vi "int32 to Hex vg.vi"(11 "number":dbl) -> (1 "Phase fied":string, 3 "E field":string)   [LabVIEW 2017]
panel:
  out "concatenated string both":string
  out "concatenated higher":string
  out "concatenated string lower":string
  out "Hex string":string
  # "RE-ENTRANT"
  # "SUBROUTINE"
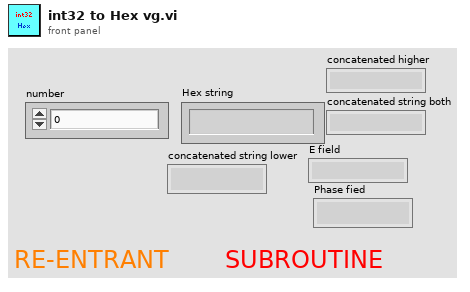
[diagram p1: front panel]
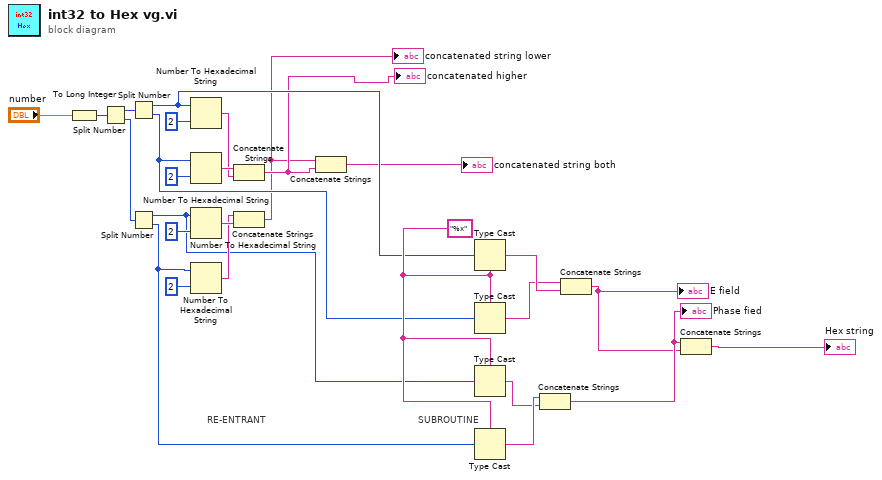
[diagram p0: block diagram]
diagram:
  w15 = "%x" ("type")
  # "SUBROUTINE"
  # "RE-ENTRANT"
  n1 = To Long Integer(number="number") -> (32bit integer=w22:i32)
  n2 = Split Number(x=w22) -> (hi(x)=w26:u16, lo(x)=w27:u16)
  n3 = Split Number(x=w26) -> (hi(x)=w12:u8, lo(x)=w13:u8)
  n4 = Split Number(x=w27) -> (hi(x)=w14:u8, lo(x)=w7:u8)
  n5 = Number To Hexadecimal String(1:i16 2 ("width (-)"), 2:w12) -> (0:w16:string)
  n6 = Number To Hexadecimal String(1:i16 2 ("width (-)"), 2:w13) -> (0:w23:string)
  n7 = Number To Hexadecimal String(1:i16 2 ("width (-)"), 2:w14) -> (0:w25:string)
  n8 = Number To Hexadecimal String(1:i16 2 ("width (-)"), 2:w7) -> (0:w24:string)
  n9 = Concatenate Strings(w23, w16) -> (w4:string)
  "concatenated higher" <- w4
  n10 = Concatenate Strings(w24, w25) -> (w3:string)
  "concatenated string lower" <- w3
  n11 = Concatenate Strings(w3, w4) -> (→"concatenated string both":string)
  n12 = Type Cast(type=w15, x=w12) -> (*(type *) &x=w9:string)
  n13 = Type Cast(type=w15, x=w13) -> (*(type *) &x=w8:string)
  n14 = Type Cast(type=w15, x=w14) -> (*(type *) &x=w10:string)
  n15 = Type Cast(type=w15, x=w7) -> (*(type *) &x=w11:string)
  n16 = Concatenate Strings(w11, w10) -> (w2:string)
  "Phase fied" <- w2
  n17 = Concatenate Strings(w8, w9) -> (w1:string)
  "E field" <- w1
  n18 = Concatenate Strings(w2, w1) -> (→"Hex string":string)
